vi "SRXConfigVoltageCompensationSingle.vi"(0 "PhoenixMotorControlDevRefIn":T6={"DeviceStatus"={"status"=FALSE, "code"=0, "source"=""}, "Type"=enum."PWM", "PWM"={"PWM Channel"=enum."PWM 1", "DeadBand"={"Name"="", "maxPositivePwm"=0, "minPositivePwm"=0, "centerPwm"=0, "maxNegativePwm"=0, "minNegativePwm"=0, "angularRange"=0}}, "CAN"={"Device Number"=0, "SetOutput VI Ref"=variant(enum8{"Percent VBus", "Current", "Speed", "Position", "Voltage"} enum."Percent VBus"), "GetOutput VI Ref"=variant(refnum<k1> refnum), "Enable VI Ref"=variant(dbl 12.0), "Disable VI Ref"=variant(enum8{"Percent VBus", "Speed", "Position", "Slave", "Unchanged / Invalid", "Voltage Compensation", "Current", "Motion Profile"} enum."Percent VBus"), "Data"=variant}, "Invert"=FALSE, "DIO PWM"={"PWM \"Enable\" Channel"=enum."Invalid", "DIOChannel"=enum."Invalid", "PWM Rate"=0.0}}, 5 "MotorConfig":T1={"CAN Address"=0, "Invert"=FALSE, "InvertSensor"=FALSE, "Unit Conversion Factor"=0.0, "Brake Mode"=enum."Override to Brake", "Reverse Limt Switch Mode"=enum."Disabled", "Forward Limt Swith Mode"=enum."Disabled", "PWM Channel"=enum."Invalid", "Motor Controller Type"=enum."Talon SRX"}, 7 "Enable Voltage Compensation?":bool, 9 "Saturation Voltage":dbl, 11 "error in (no error)":errorcluster) -> (4 "PhoenixMotorControlDevRefOut":T6={"DeviceStatus"={"status"=FALSE, "code"=0, "source"=""}, "Type"=enum."PWM", "PWM"={"PWM Channel"=enum."PWM 1", "DeadBand"={"Name"="", "maxPositivePwm"=0, "minPositivePwm"=0, "centerPwm"=0, "maxNegativePwm"=0, "minNegativePwm"=0, "angularRange"=0}}, "CAN"={"Device Number"=0, "SetOutput VI Ref"=variant(enum8{"Percent VBus", "Current", "Speed", "Position", "Voltage"} enum."Percent VBus"), "GetOutput VI Ref"=variant(refnum<k1> refnum), "Enable VI Ref"=variant(dbl 12.0), "Disable VI Ref"=variant(enum8{"Percent VBus", "Speed", "Position", "Slave", "Unchanged / Invalid", "Voltage Compensation", "Current", "Motion Profile"} enum."Percent VBus"), "Data"=variant}, "Invert"=FALSE, "DIO PWM"={"PWM \"Enable\" Channel"=enum."Invalid", "DIOChannel"=enum."Invalid", "PWM Rate"=0.0}}, 15 "error out":errorcluster)   [LabVIEW 2017, in "ArgosLib.lvlib"]
uses:
  ArgosLib.lvlib
  <vilib>/Rock Robotics/WPI/MotorControl/WPI_MotorControlDeviceRef.ctl
  <vilib>/Rock Robotics/WPI/MotorControl/WPI_MotorControlType.ctl
  <vilib>/Rock Robotics/SystemInterfaces/DIO/FPGA_DIOPWMChannel.ctl
  <vilib>/Rock Robotics/WPI/PWM/WPI_PWMDeadband.ctl
  <vilib>/Rock Robotics/SystemInterfaces/DIO/FPGA_DIOChannel.ctl
  Config/ConfigComponents/TypeDefs/Config_Motor.ctl
  <vilib>/Rock Robotics/WPI/ThirdParty/Phoenix-LabVIEW/Motor Controller/Controls/CTRE_Phoenix_MotorControl_NeutralMode.ctl
  <vilib>/Rock Robotics/WPI/ThirdParty/Phoenix-LabVIEW/Motor Controller/Controls/CTRE_Phoenix_MotorControl_LimitSwitchNormal.ctl
  Config/ConfigComponents/TypeDefs/Config_MotorCtrlType.ctl
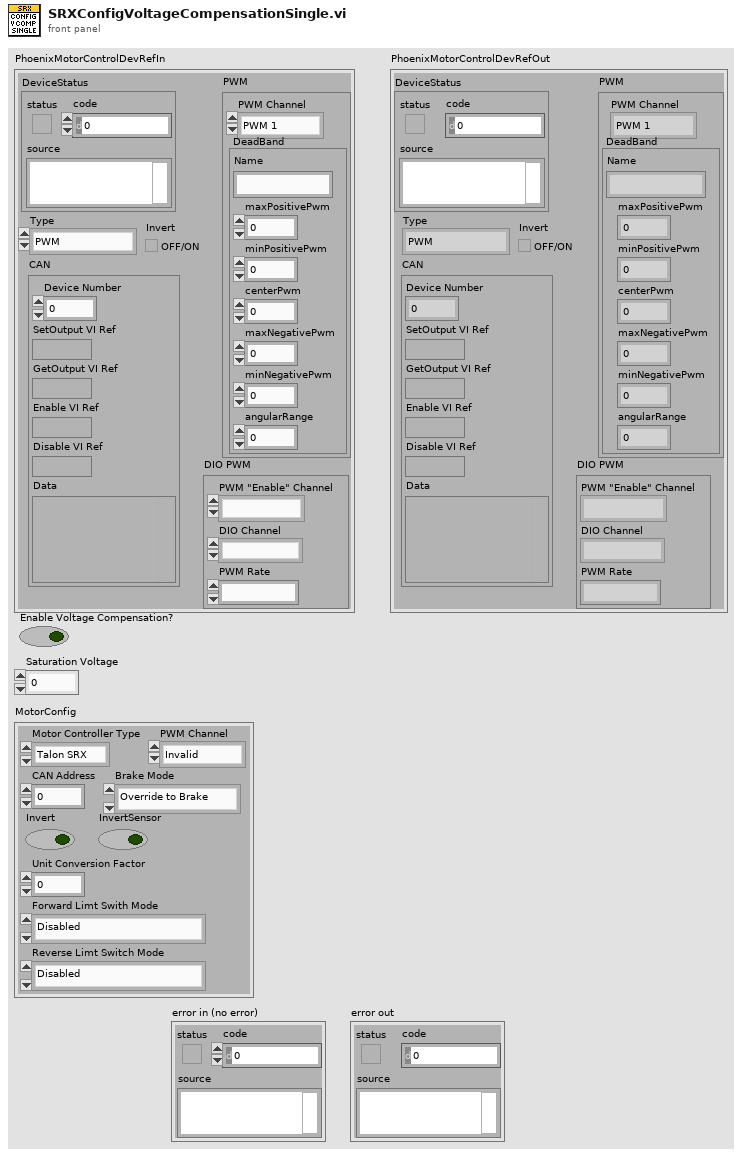
[diagram p1: front panel]
types:
  T1 = typedef "ArgosLib.lvlib/Config_Motor.ctl" = cluster{"CAN Address":u8, "Invert":bool, "InvertSensor":bool, "Unit Conversion Factor":dbl, "Brake Mode":T2, "Reverse Limt Switch Mode":T3, "Forward Limt Swith Mode":T3, "PWM Channel":T4, "Motor Controller Type":T5}
  T2 = typedef "CTRE_Phoenix_MotorControl_NeutralMode.ctl" = enum8{"EEPROMSetting", "Override to Coast", "Override to Brake"}
  T3 = typedef "CTRE_Phoenix_MotorControl_LimitSwitchNormal.ctl" = enum16{"Normally Open", "Normally Closed", "Disabled"}
  T4 = typedef "FPGA_DIOPWMChannel.ctl" = enum8{"PWM 0", "PWM 1", "PWM 2", "PWM 3", "PWM 4", "PWM 5", "PWM 6", "PWM 7", "PWM 8", "PWM 9", "PWM MXP 0", "PWM MXP 1", "PWM MXP 2", "PWM MXP 3", "PWM MXP 4", "PWM MXP 5", "PWM MXP 6", "PWM MXP 7", "PWM MXP 8", "PWM MXP 9", "Invalid"}
  T5 = typedef "ArgosLib.lvlib/Config_MotorCtrlType.ctl" = enum16{"Disabled", "Talon SRX", "Talon SR"}
  T6 = typedef "WPI_MotorControlDeviceRef.ctl" = cluster{"DeviceStatus":errorcluster, "Type":T7, "PWM":cluster{"PWM Channel":T4, "DeadBand":T8}, "CAN":cluster{"Device Number":u8, "SetOutput VI Ref":variant, "GetOutput VI Ref":variant, "Enable VI Ref":variant, "Disable VI Ref":variant, "Data":variant}, "Invert":bool, "DIO PWM":cluster{"PWM \"Enable\" Channel":T4, "DIOChannel":T9, "PWM Rate":dbl}}
  T7 = typedef "WPI_MotorControlType.ctl" = enum16{"PWM", "CAN", "DIO PWM"}
  T8 = typedef "WPI_PWMDeadband.ctl" = cluster{"Name":string, "maxPositivePwm":i32, "minPositivePwm":i32, "centerPwm":i32, "maxNegativePwm":i32, "minNegativePwm":i32, "angularRange":u16}
  T9 = typedef "FPGA_DIOChannel.ctl" = enum8{"DIO 0", "DIO 1", "DIO 2", "DIO 3", "DIO 4", "DIO 5", "DIO 6", "DIO 7", "DIO 8", "DIO 9", "DIO MXP 0", "DIO MXP 1", "DIO MXP 2", "DIO MXP 3", "DIO MXP 4", "DIO MXP 5", "DIO MXP 6", "DIO MXP 7", "DIO MXP 8", "DIO MXP 9", "DIO MXP 10", "DIO MXP 11", "DIO MXP 12", "DIO MXP 13", "DIO MXP 14", "DIO MXP 15", "SPI Port CS1", "SPI Port CS2", "SPI Port CS3", "SPI Port MISO", "SPI Port MOSI", "Invalid"}
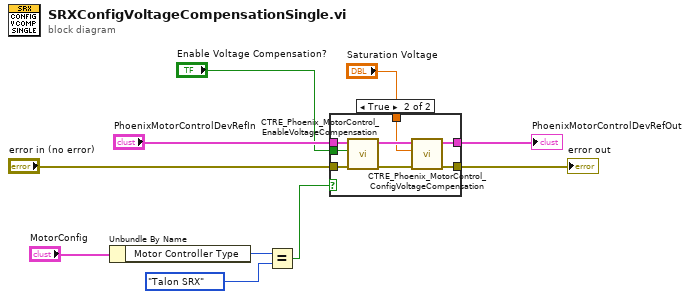
[diagram p0: block diagram]
diagram:
  n1 = Unbundle By Name("MotorConfig") -> ("Motor Controller Type"=w3:T5)
  n2 = Equal?(x=w3, y=Config_MotorCtrlType."Talon SRX") -> (x = y?=w1:bool)
  n3 = case shown="True" w1 {
    tunnel: "PhoenixMotorControlDevRefIn" -> [w12 w18]
    tunnel: [w12 w17] -> w9
    tunnel: "Enable Voltage Compensation?" -> [_ w16]
    tunnel: "Saturation Voltage" -> [_ w15]
    tunnel: "error in (no error)" -> [w11 w14]
    tunnel: [w11 w13] -> w5
    frame False {
    }
    frame True {
      n4 = call <vilib>:"CTRE_Phoenix_MotorControl_EnableVoltageCompensation.vi"("error in (no error)"=w14, "Enable Voltage Compensation?"=w16, "PhoenixMotorControlDevRef"=w18) -> ("error out"=w19:errorcluster, "PhoenixMotorControlDevRef"=w20:T6)  [unwired: 7 in]
      n5 = call <vilib>:"CTRE_Phoenix_MotorControl_ConfigVoltageCompensation.vi"("error in (no error)"=w19, "Saturation Voltage"=w15, "PhoenixMotorControlDevRef"=w20) -> ("error out"=w13:errorcluster, "PhoenixMotorControlDevRef"=w17:T6)  [unwired: 7 in]
    }
  }
  "PhoenixMotorControlDevRefOut" <- w9
  "error out" <- w5
